vi "add_standard_info.vi"(8 "error in (no error)":errorcluster, 10 "data array":string[](array[string]), 11 "Analysis in":refnum<class "Analysis.lvclass">) -> (0 "error out":errorcluster, 2 "data array out":string[](array[string]), 3 "Analysis out":refnum<class "Analysis.lvclass">)   [LabVIEW 2015]
doc: "input is the data array from the text file.\nThe VI searches forthe standard info and writes the data into the AnalysisObject"
uses:
  MSControl/Classes/Analysis/Analysis.lvclass
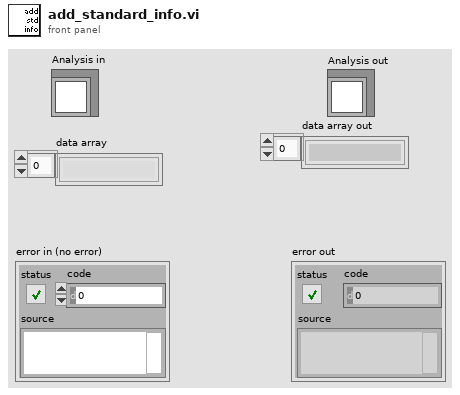
[diagram p1: front panel]
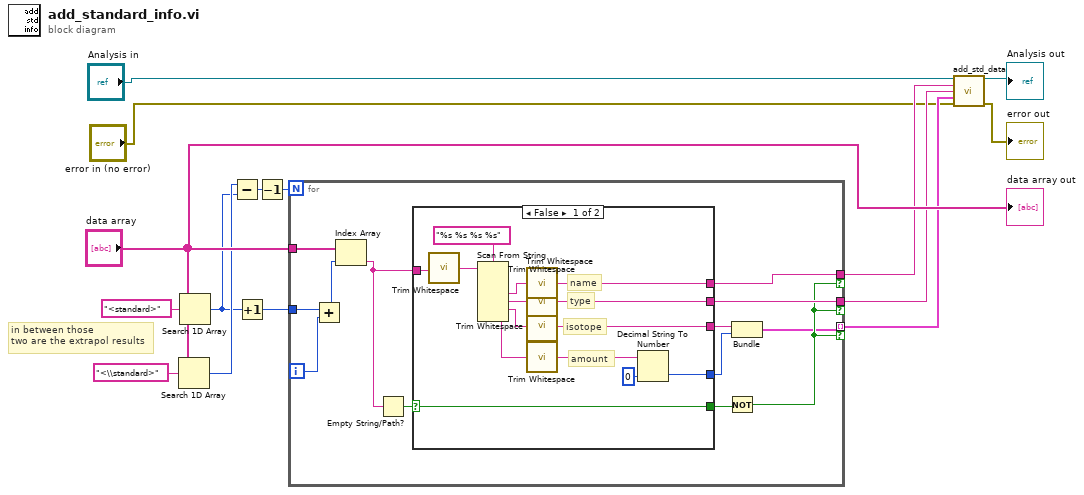
[diagram p0: block diagram]
diagram:
  # "in between those\ntwo are the extrapol results"
  n1 = Search 1D Array(1D array="data array", element="<\\standard>") -> (index of element=w12:i32)  [unwired: 1 in]
  n2 = Search 1D Array(1D array="data array", element="<standard>") -> (index of element=w10:i32)  [unwired: 1 in]
  n3 = Subtract(x=w12, y=w10) -> (x-y=w9:i32)
  n4 = Increment(x=w10) -> (x+1=w11:i32)
  n5 = Decrement(x=w9) -> (x-1=w8:i32)
  n6 = for {
    N: w8 -> [_]
    tunnel: "data array" -> [w28]
    tunnel: w11 -> [w27]
    tunnel: [w21] -> w6 if=w19
    tunnel: [w20] -> w5 if=w19
    tunnel: [w16] -> w7 mode=indexing if=w19
    i -> [w26]
    n7 = Add(x=w27, y=w26) -> (x+y=w25:i32)
    n8 = Index Array(array=w28, index=w25) -> (element=w24:string)
    n9 = Empty String/Path?(string/path=w24) -> (empty?=w23:bool)
    n10 = case shown="False" w23 {
      selector: w23 -> [w39 w43]
      tunnel: w24 -> [w40 _]
      tunnel: [w39 w43] -> w22
      tunnel: [w34 _] -> w21
      tunnel: [w33 _] -> w20
      tunnel: [w32 _] -> w18
      tunnel: [w29 _] -> w17
      frame False {
        # "amount"
        # "isotope"
        # "type"
        # "name"
        n11 = call <vilib>:"Trim Whitespace.vi"("string"=w40) -> ("trimmed string"=w42:string)  [unwired: 1 in]
        n12 = Scan From String(format string="%s %s %s %s", input string=w42) -> (output 1=w38:string, output 2=w37:string, output 3=w36:string, output 4=w35:string)  [unwired: 6 in, 3 out]
        n13 = call <vilib>:"Trim Whitespace.vi"("string"=w38) -> ("trimmed string"=w34:string)  [unwired: 1 in]
        n14 = call <vilib>:"Trim Whitespace.vi"("string"=w37) -> ("trimmed string"=w33:string)  [unwired: 1 in]
        n15 = call <vilib>:"Trim Whitespace.vi"("string"=w36) -> ("trimmed string"=w32:string)  [unwired: 1 in]
        n16 = call <vilib>:"Trim Whitespace.vi"("string"=w35) -> ("trimmed string"=w30:string)  [unwired: 1 in]
        n17 = Decimal String To Number(string=w30, default (0L)=i64 0 ("default (0 I32)")) -> (number=w29:i64)  [unwired: 1 in, 1 out]
      }
      frame True {
      }
    }
    n18 = Not(x=w22) -> (.not. x?=w19:bool)
    n19 = Bundle("trimmed string"=w18, w17) -> (w16:cluster{"trimmed string":string, i64})  [unwired: 1 in]
  }
  n20 = call "add_std_data.vi"("Analysis in"="Analysis in", "standard_name"=w6, "standard_type"=w5, "Isotope Table"=w7, "error in (no error)"="error in (no error)") -> ("Analysis out"=→"Analysis out":refnum<class "Analysis.lvclass">, "error out"=→"error out":errorcluster)  [unwired: 9 in]
  "data array out" <- "data array"
